vi "view_full_data.vi"(9 "data":dbl[][][](array[numeric]), 11 "wavelength":dbl[](array[numeric])) -> ()   [LabVIEW 2019]
panel:
  out "size(s)":i32[](array[numeric])
  out "Intensity Graph 2":dbl[][](graph)
  out "XY Graph 2":cluster{"data":dbl[], i32[]}(graph)
  out "XY Graph":cluster{"data":dbl[], i32[]}(graph)
  out "Intensity Graph":dbl[][](graph)
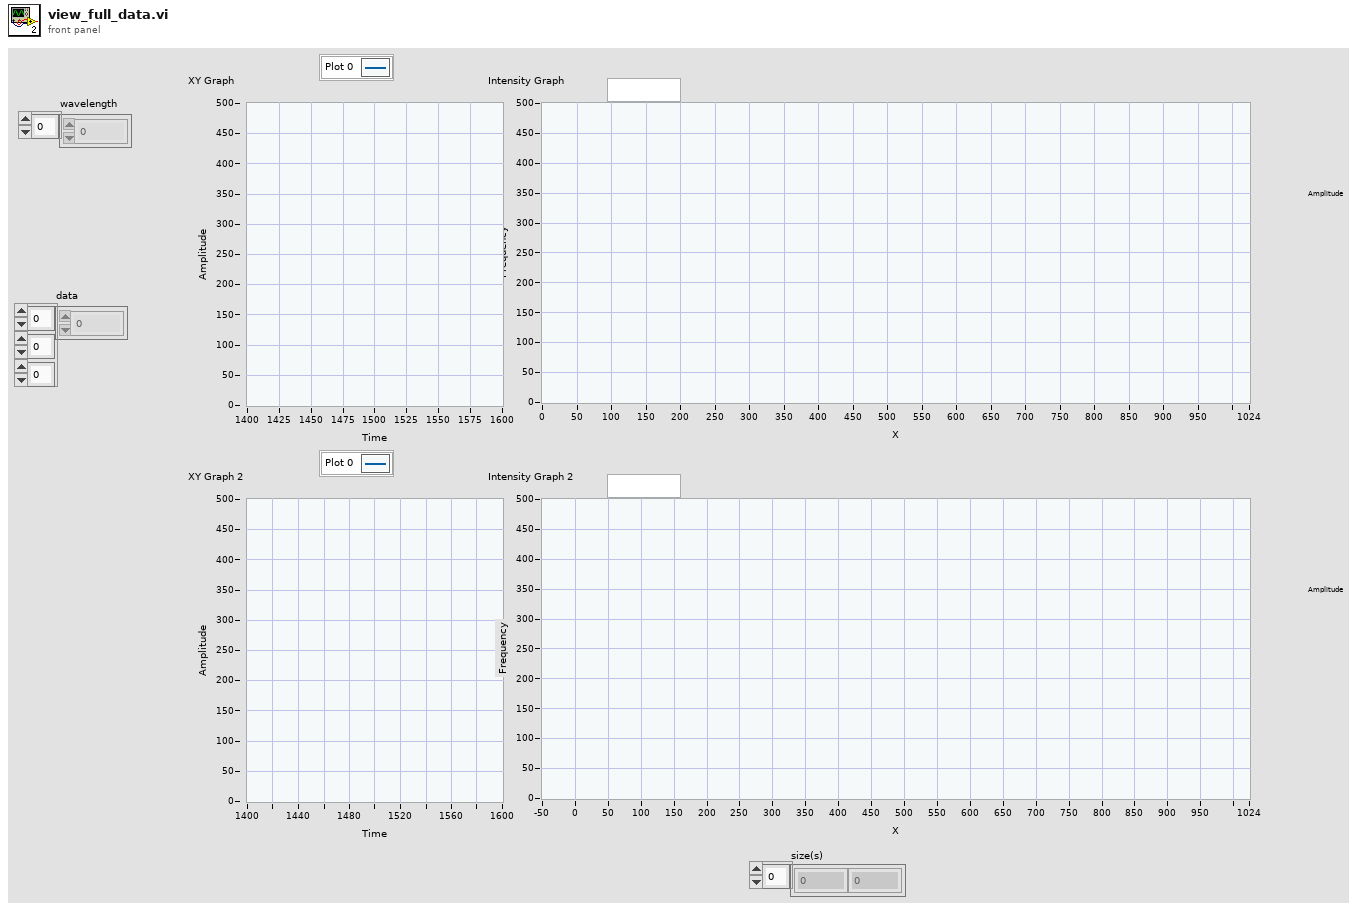
[diagram p1: front panel]
types:
  T1 = enum32{"Invalid", "Standard", "Closed", "Hidden", "Minimized", "Maximized"}
  T2 = typedef "LVCursorListTypeDef.ctl" = cluster{"Name":string, "Color":u32, "Style":u8, "Point Style":u8, "Name Visible":bool, "Allow Drag":bool, "Cursor Mode":u32, "Plot":i32, "Index":i32, "Position":cluster{"X":dbl, "Y":dbl}, "X Scale":u32, "Y Scale":u32, "Watch Plots":i32[], "Watch All Plots":bool, "Plot Area":i32, "Label Offset":cluster{"X":dbl, "Y":dbl}}[]
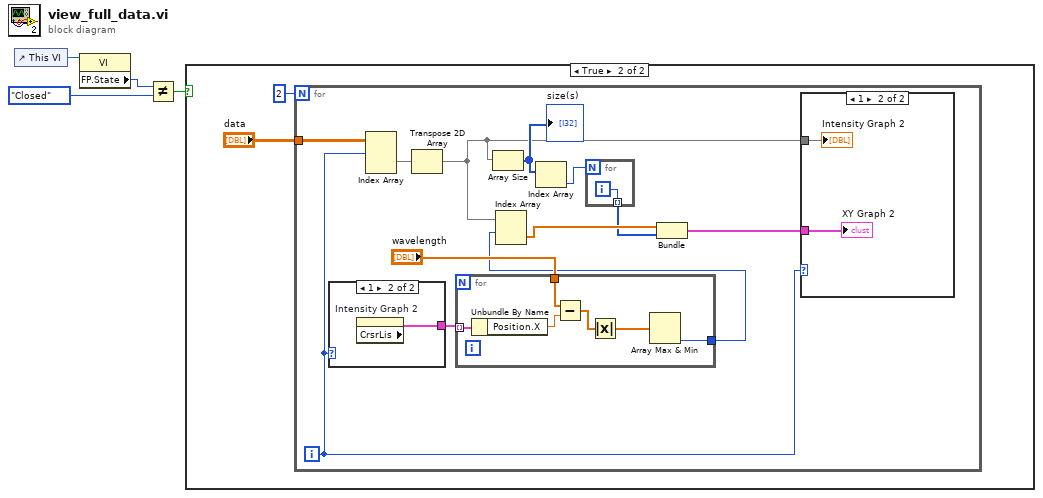
[diagram p0: block diagram]
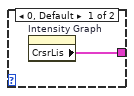
[diagram p3: hidden frame]
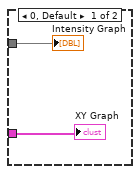
[diagram p4: hidden frame]
diagram:
  n1 = control-ref of="This VI"() -> (w4:refnum<vi>)
  n2 = property class="VI"(reference=w4) -> ("FP.State"=w3:T1)  [unwired: 1 in, 2 out]
  n3 = Not Equal?(x=w3, y=T1."Closed") -> (x != y?=w1:bool)
  n4 = case shown="True" w1 {
    frame False {
    }
    frame True {
      n5 = for {
        N: 2 -> [_]
        tunnel: "data" -> [w11]
        i -> [w8]
        n6 = case shown="1" w8 {
          tunnel: [w19 w20] -> w7
          frame 0, Default {
            n7 = property on="Intensity Graph" class="IntGraph (strict)"() -> ("CrsrLis"=w19:T2)  [unwired: 2 in, 2 out]
          }
          frame 1 {
            n8 = property on="Intensity Graph 2" class="IntGraph (strict)"() -> ("CrsrLis"=w20:T2)  [unwired: 2 in, 2 out]
          }
        }
        n9 = Index Array(array=w11, index (dim 0)=w8) -> (element=w10:dbl[][])  [unwired: 2 in]
        n10 = Transpose 2D Array(2D array=w10) -> (transposed array=w9:dbl[][])
        n11 = for {
          tunnel: "wavelength" -> [w31]
          tunnel: w7 -> [w28] mode=indexing
          tunnel: [w26] -> w16
          n12 = Unbundle By Name(w28) -> ("Position.X"=w30:dbl)
          n13 = Subtract(x=w31, y=w30) -> (x-y=w29:dbl[])
          n14 = Absolute Value(x=w29) -> (abs(x)=w27:dbl[])
          n15 = Array Max & Min(array=w27) -> (min index (indices)=w26:i32)  [unwired: 3 out]
        }
        n16 = Array Size(array=w9) -> (size(s)=w14:i32[])
        "size(s)" <- w14
        n17 = Index Array(array=w9, index (row)=w16) -> (element=w18:dbl[])  [unwired: 1 in]
        n18 = Index Array(array=w14) -> (element=w13:i32)  [unwired: 1 in]
        n19 = for {
          N: w13 -> [_]
          tunnel: [w25] -> w15 mode=indexing
          i -> [w25]
        }
        n20 = Bundle(w18, w15) -> (w12:cluster{dbl[], i32[]})  [unwired: 1 in]
        n21 = case shown="1" w8 {
          tunnel: w12 -> [w22 w23]
          tunnel: w9 -> [w21 w24]
          frame 0, Default {
            "XY Graph" <- w22
            "Intensity Graph" <- w21
          }
          frame 1 {
            "XY Graph 2" <- w23
            "Intensity Graph 2" <- w24
          }
        }
      }
    }
  }
